vi "Begin.vi"(11 "Image Size":T1=enum."320x240") -> (0 "error out":errorcluster)   [LabVIEW 2012]
doc: "Called before other user functions, this VI is expected to open initial I/O refnums, load in file data, and do all program initialization. Notice that the <B>error out</B> terminal is simply used for data flow. Wiring it to other structures or subVIs ensures that this VI runs first."
uses:
  <vilib>/Rock Robotics/WPI/Camera/WPI_CameraImageSize.ctl
  <vilib>/Rock Robotics/WPI/DriverStation/WPI_DriverStationRobotMode2.ctl
  <vilib>/Rock Robotics/SystemInterfaces/DIO/FPGA_DIOPWMChannel.ctl
  <vilib>/Rock Robotics/WPI/Joystick/WPI_JoystickDeviceEnum.ctl
  <vilib>/Rock Robotics/SystemInterfaces/Typedef/FPGA_TypedefDigitalModule.ctl
  <vilib>/Rock Robotics/WPI/Relay/WPI_RelayDirection.ctl
  <vilib>/Rock Robotics/SystemInterfaces/DIO/FPGA_DIORelayChannel.ctl
  <vilib>/Rock Robotics/SystemInterfaces/AI/FPGA_AIChannel.ctl
  <vilib>/Rock Robotics/SystemInterfaces/AI/FPGA_AIGyroChannel.ctl
  <vilib>/Rock Robotics/SystemInterfaces/DIO/FPGA_DIOChannel.ctl
  <vilib>/Rock Robotics/WPI/Camera/WPI_CameraFrameRate.ctl
  Robot Global Data.vi
  <vilib>/Rock Robotics/WPI/MotorControl/WPI_MotorControlOpen Victor.vi
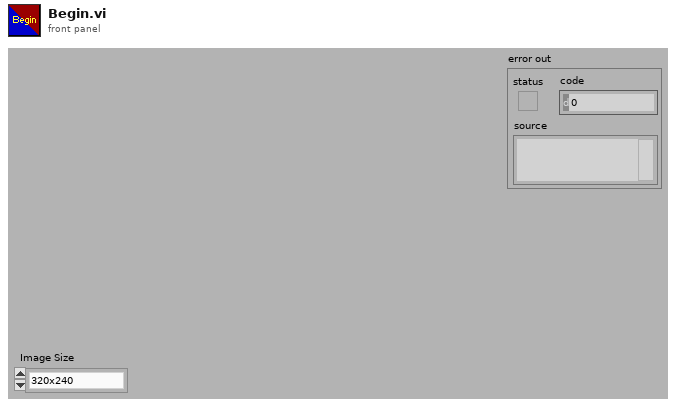
[diagram p1: front panel]
types:
  T1 = typedef "WPI_CameraImageSize.ctl" = enum16{"640x480", "320x240", "160x120"}
  T2 = typedef "FPGA_DIOChannel.ctl" = enum8{"DIO 1", "DIO 2", "DIO 3", "DIO 4", "DIO 5", "DIO 6", "DIO 7", "DIO 8", "DIO 9", "DIO 10", "DIO 11", "DIO 12", "DIO 13", "DIO 14", "Invalid"}
  T3 = typedef "FPGA_TypedefDigitalModule.ctl" = enum16{"Digital Module 1", "Digital Module 2"}
  T4 = typedef "FPGA_DIOPWMChannel.ctl" = enum8{"PWM 1", "PWM 2", "PWM 3", "PWM 4", "PWM 5", "PWM 6", "PWM 7", "PWM 8", "PWM 9", "PWM 10", "Invalid"}
  T5 = typedef "FPGA_DIORelayChannel.ctl" = enum8{"Relay 1", "Relay 2", "Relay 3", "Relay 4", "Relay 5", "Relay 6", "Relay 7", "Relay 8", "Invalid"}
  T6 = typedef "WPI_RelayDirection.ctl" = enum16{"Both directions", "Forward only", "Reverse only"}
  T7 = typedef "WPI_CameraFrameRate.ctl" = u32
  T8 = typedef "FPGA_AIChannel.ctl" = enum8{"AI 1", "AI 2", "AI 3", "AI 4", "AI 5", "AI 6", "AI 7", "AI 8", "Invalid"}
  T9 = typedef "FPGA_AIGyroChannel.ctl" = enum8{"AI 1", "AI 2", "Invalid"}
  T10 = typedef "WPI_JoystickDeviceEnum.ctl" = enum16{"USB 1", "USB 2", "USB 3", "USB 4", "Kinect 1", "Kinect 2"}
  T11 = typedef "WPI_DriverStationRobotMode2.ctl" = enum16{"Autonomous Disabled", "Autonomous Enabled", "Teleop Disabled", "Teleop Enabled", "Timeout", "Finish", "Test Disabled", "Test Enabled"}
  T12 = typedef "WPI_RelayDevRef.ctl" = cluster{"DevStatus":errorcluster, "Relay Channel":T5, "Digital Module":T3, "Relay Direction":T6}
  T13 = typedef "WPI_MotorControlDeviceRef.ctl" = cluster{"DeviceStatus":errorcluster, "Type":enum16{"PWM", "CAN"}, "PWM":cluster{"Digital Module":T3, "PWM Channel":T4, "DeadBand":T14}, "CAN":cluster{"Device Number":u8, "Control Mode":T15, "Semaphore":T16, "Max Vout":dbl}, "Invert":bool, "TransformRef":T17, "InvTransformRef":T17}
  T14 = typedef "WPI_PWMDeadband.ctl" = cluster{"Name":string, "maxPositivePwm":i32, "minPositivePwm":i32, "centerPwm":i32, "maxNegativePwm":i32, "minNegativePwm":i32, "angularRange":u16}
  T15 = typedef "WPI_CANJaguar_ControlMode.ctl" = enum8{"Percent VBus", "Current", "Speed", "Position", "Voltage"}
  T16 = typedef "Semaphore RefNum" = refnum<k1>
  T17 = typedef "WPI_PWMTransform_ConPane.ctl" = refnum<vi>
  T18 = typedef "WPI_JoystickDevRef.ctl" = cluster{"Device":T10}
  T19 = typedef "WPI_CameraDevRef.ctl" = cluster{"Camera Address":string, "CameraStatus":errorcluster, "Acquire Image Notifier":refnum<notifier>}
  T20 = typedef "WPI_ServoDeviceRef.ctl" = cluster{"DeviceStatus":errorcluster, "Digital Module":T3, "PWM Channel":T4, "DeadBand":T14}
  T21 = typedef "WPI_AnalogChannelDevRef.ctl" = cluster{"DevStatus":errorcluster, "Analog Module":T22, "Analog Channel":T8}
  T22 = typedef "FPGA_TypedefAnalogModule.ctl" = enum16{"Analog Module 1", "Analog Module 2"}
  T23 = typedef "WPI_DigitalInputDevRef.ctl" = cluster{"DevStatus":errorcluster, "DIO Channel":T2, "Digital Module":T3}
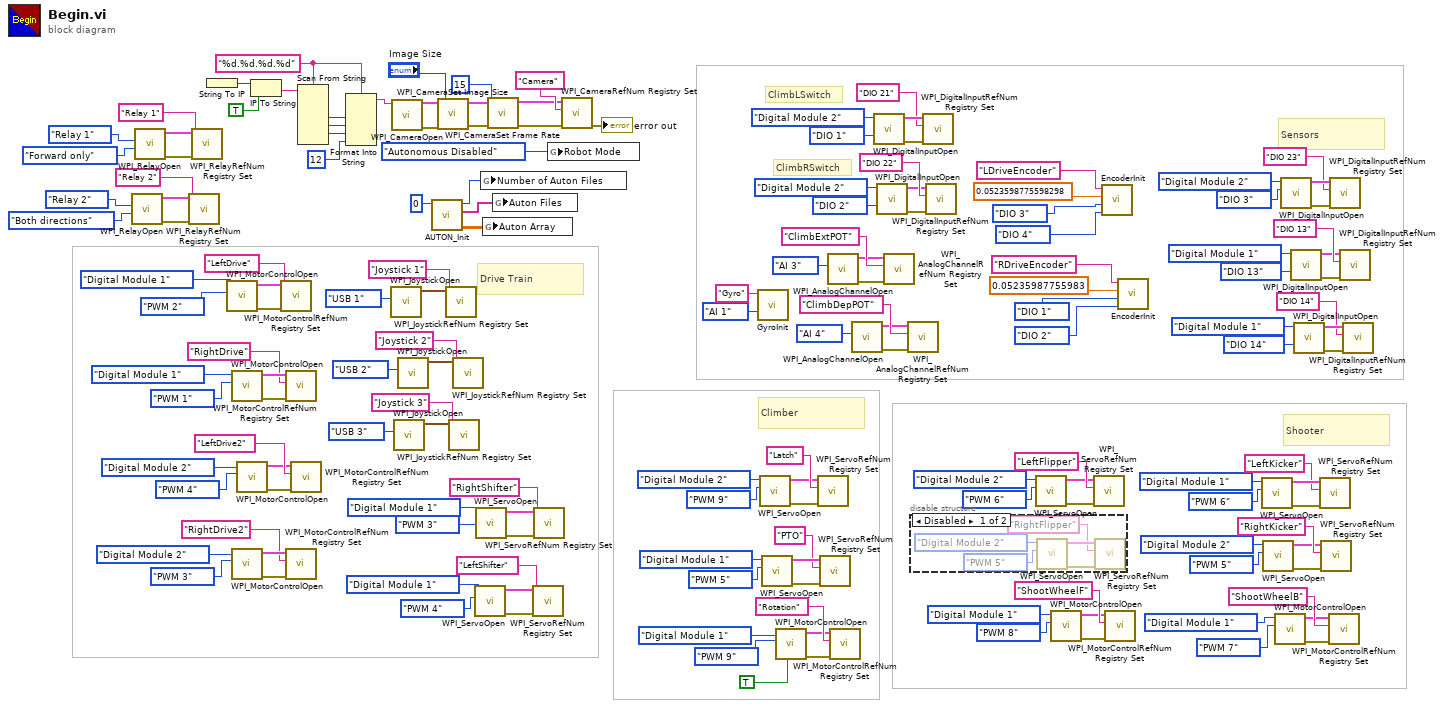
[diagram p0: block diagram]
diagram:
  w70 = "%d.%d.%d.%d" ("format string")
  # "ClimbRSwitch"
  # "ClimbLSwitch"
  # "Shooter"
  # "Drive Train"
  # "Climber"
  # "Sensors"
  n1 = call <vilib>:"WPI_RelayOpen.vi"("Relay Direction"=WPI_RelayDirection."Both directions", "Relay Channel"=FPGA_DIORelayChannel."Relay 2") -> ("error out"=w119:errorcluster, "RelayDevRef"=w120:T12)  [unwired: 8 in]
  n2 = call <vilib>:"WPI_RelayOpen.vi"("Relay Direction"=WPI_RelayDirection."Forward only", "Relay Channel"=FPGA_DIORelayChannel."Relay 1") -> ("error out"=w60:errorcluster, "RelayDevRef"=w59:T12)  [unwired: 8 in]
  n3 = call <vilib>:"WPI_RelayRefNum Registry Set.vi"("error in (no error)"=w119, "refnum name"="Relay 2", "RelayDevRef"=w120) -> ()  [unwired: 7 in, 2 out]
  n4 = call <vilib>:"WPI_RelayRefNum Registry Set.vi"("error in (no error)"=w60, "refnum name"="Relay 1", "RelayDevRef"=w59) -> ()  [unwired: 7 in, 2 out]
  n5 = String To IP() -> (0:w77:u32)  [unwired: 1 in]
  n6 = call-poly <vilib>:"WPI_MotorControlOpen.vi"("PWM Channel"=FPGA_DIOPWMChannel."PWM 2", "Digital Module (Module 1)"=FPGA_TypedefDigitalModule."Digital Module 1") -> ("error out"=w145:errorcluster, "MotorControlDeviceRef"=w146:T13)  [unwired: 8 in]
  n7 = call-poly <vilib>:"WPI_MotorControlOpen.vi"("PWM Channel"=FPGA_DIOPWMChannel."PWM 1", "Digital Module (Module 1)"=FPGA_TypedefDigitalModule."Digital Module 1") -> ("error out"=w152:errorcluster, "MotorControlDeviceRef"=w151:T13)  [unwired: 8 in]
  n8 = call-poly <vilib>:"WPI_MotorControlOpen.vi"("PWM Channel"=FPGA_DIOPWMChannel."PWM 3", "Digital Module (Module 1)"=FPGA_TypedefDigitalModule."Digital Module 2") -> ("error out"=w134:errorcluster, "MotorControlDeviceRef"=w133:T13)  [unwired: 8 in]
  n9 = call-poly <vilib>:"WPI_MotorControlOpen.vi"("PWM Channel"=FPGA_DIOPWMChannel."PWM 4", "Digital Module (Module 1)"=FPGA_TypedefDigitalModule."Digital Module 2") -> ("error out"=w125:errorcluster, "MotorControlDeviceRef"=w126:T13)  [unwired: 8 in]
  n10 = IP To String(1:TRUE ("dot notation? (F)"), 2:w77) -> (0:w75:string)
  n11 = call <vilib>:"WPI_MotorControlRefNum Registry Set.vi"("error in (no error)"=w145, "refnum name"="LeftDrive", "MotorControlDevRef"=w146) -> ()  [unwired: 7 in, 2 out]
  n12 = call <vilib>:"WPI_MotorControlRefNum Registry Set.vi"("error in (no error)"=w152, "refnum name"="RightDrive", "MotorControlDevRef"=w151) -> ()  [unwired: 7 in, 2 out]
  n13 = call <vilib>:"WPI_MotorControlRefNum Registry Set.vi"("error in (no error)"=w134, "refnum name"="RightDrive2", "MotorControlDevRef"=w133) -> ()  [unwired: 7 in, 2 out]
  n14 = call <vilib>:"WPI_MotorControlRefNum Registry Set.vi"("error in (no error)"=w125, "refnum name"="LeftDrive2", "MotorControlDevRef"=w126) -> ()  [unwired: 7 in, 2 out]
  n15 = Scan From String(format string=w70, input string=w75) -> (output 1=w74:i32, output 2=w73:i32, output 3=w72:i32)  [unwired: 7 in, 3 out]
  n16 = Format Into String(format string=w70, w74, w73, w72, 12 ("Compression")) -> (resulting string=w69:string)  [unwired: 2 in, 1 out]
  n17 = call <vilib>:"WPI_JoystickOpen.vi"("JoystickDevice"=WPI_JoystickDeviceEnum."USB 1") -> ("JoystickDevRef"=w136:T18)  [unwired: 10 in]
  n18 = call <vilib>:"WPI_CameraOpen.vi"("Camera Address"=w69) -> ("error out"=w68:errorcluster, "CameraDevRef"=w67:T19)  [unwired: 1 in, 8 out]
  n19 = call <vilib>:"WPI_JoystickOpen.vi"("JoystickDevice"=WPI_JoystickDeviceEnum."USB 3") -> ("JoystickDevRef"=w142:T18)  [unwired: 10 in]
  n20 = call <vilib>:"WPI_JoystickOpen.vi"("JoystickDevice"=WPI_JoystickDeviceEnum."USB 2") -> ("JoystickDevRef"=w141:T18)  [unwired: 10 in]
  n21 = call "AUTON_Init.vi"("Default File"=0) -> ("Auton Array"=w153:dbl[][], "Auton Files"=w154:string[], "Number of Auton Files"=w155:i64)  [unwired: 8 in]
  n22 = call <vilib>:"WPI_CameraSet Image Size.vi"("error in (no error)"=w68, "Image Size"="Image Size", "CameraDevRef"=w67) -> ("error out"=w65:errorcluster, "CameraDevRef Out"=w66:T19)  [unwired: 7 out]
  n23 = call <vilib>:"WPI_JoystickRefNum Registry Set.vi"("refnum name"="Joystick 1", "JoystickDevRef"=w136) -> ()  [unwired: 8 in, 2 out]
  n24 = call <vilib>:"WPI_JoystickRefNum Registry Set.vi"("refnum name"="Joystick 3", "JoystickDevRef"=w142) -> ()  [unwired: 8 in, 2 out]
  n25 = call <vilib>:"WPI_JoystickRefNum Registry Set.vi"("refnum name"="Joystick 2", "JoystickDevRef"=w141) -> ()  [unwired: 8 in, 2 out]
  n26 = call <vilib>:"WPI_ServoOpen.vi"("PWM Channel"=FPGA_DIOPWMChannel."PWM 4", "Digital Module (Module 1)"=FPGA_TypedefDigitalModule."Digital Module 1") -> ("error out"=w118:errorcluster, "ServoDeviceRef"=w111:T20)  [unwired: 8 in]
  n27 = call <vilib>:"WPI_ServoOpen.vi"("PWM Channel"=FPGA_DIOPWMChannel."PWM 3", "Digital Module (Module 1)"=FPGA_TypedefDigitalModule."Digital Module 1") -> ("error out"=w117:errorcluster, "ServoDeviceRef"=w116:T20)  [unwired: 8 in]
  n28 = global write "Robot Global Data.vi" "Number of Auton Files"(w155) -> ()
  n29 = global write "Robot Global Data.vi" "Auton Array"(w153) -> ()
  n30 = call <vilib>:"WPI_CameraSet Frame Rate.vi"("error in (no error)"=w65, "Frame Rate (fps)"=T7 15, "CameraDevRef"=w66) -> ("error out"=w64:errorcluster, "CameraDevRef Out"=w63:T19)  [unwired: 7 out]
  n31 = global write "Robot Global Data.vi" "Auton Files"(w154) -> ()
  n32 = call <vilib>:"WPI_ServoRefNum Registry Set.vi"("error in (no error)"=w118, "refnum name"="LeftShifter", "ServoDeviceRef"=w111) -> ()  [unwired: 7 in, 2 out]
  n33 = call <vilib>:"WPI_ServoRefNum Registry Set.vi"("error in (no error)"=w117, "refnum name"="RightShifter", "ServoDeviceRef"=w116) -> ()  [unwired: 7 in, 2 out]
  n34 = global write "Robot Global Data.vi" "Robot Mode"(WPI_DriverStationRobotMode2."Autonomous Disabled" ("Robot Mode")) -> ()
  n35 = call <vilib>:"WPI_CameraRefNum Registry Set.vi"("error in (no error)"=w64, "refnum name"="Camera", "CameraDevRef"=w63) -> ("error out"=→"error out":errorcluster)  [unwired: 8 out]
  n36 = call "GyroInit.vi"("refnum name"="Gyro", "Analog Channel"=FPGA_AIGyroChannel."AI 1") -> ()  [unwired: 8 in]
  n37 = call <vilib>:"WPI_ServoOpen.vi"("PWM Channel"=FPGA_DIOPWMChannel."PWM 9", "Digital Module (Module 1)"=FPGA_TypedefDigitalModule."Digital Module 2") -> ("error out"=w52:errorcluster, "ServoDeviceRef"=w53:T20)  [unwired: 8 in]
  n38 = call <vilib>:"WPI_ServoOpen.vi"("PWM Channel"=FPGA_DIOPWMChannel."PWM 5", "Digital Module (Module 1)"=FPGA_TypedefDigitalModule."Digital Module 1") -> ("error out"=w96:errorcluster, "ServoDeviceRef"=w95:T20)  [unwired: 8 in]
  n39 = call-poly <vilib>:"WPI_MotorControlOpen.vi"("Invert"=TRUE, "PWM Channel"=FPGA_DIOPWMChannel."PWM 9", "Digital Module (Module 1)"=FPGA_TypedefDigitalModule."Digital Module 1") -> ("error out"=w101:errorcluster, "MotorControlDeviceRef"=w100:T13)  [unwired: 7 in]
  n40 = call <vilib>:"WPI_ServoRefNum Registry Set.vi"("error in (no error)"=w52, "refnum name"="Latch", "ServoDeviceRef"=w53) -> ()  [unwired: 7 in, 2 out]
  n41 = call <vilib>:"WPI_ServoRefNum Registry Set.vi"("error in (no error)"=w96, "refnum name"="PTO", "ServoDeviceRef"=w95) -> ()  [unwired: 7 in, 2 out]
  n42 = call <vilib>:"WPI_AnalogChannelOpen.vi"("Analog Channel"=FPGA_AIChannel."AI 3") -> ("error out"=w80:errorcluster, "AIDeviceRef"=w81:T21)  [unwired: 9 in]
  n43 = call <vilib>:"WPI_MotorControlRefNum Registry Set.vi"("error in (no error)"=w101, "refnum name"="Rotation", "MotorControlDevRef"=w100) -> ()  [unwired: 7 in, 2 out]
  n44 = call <vilib>:"WPI_AnalogChannelOpen.vi"("Analog Channel"=FPGA_AIChannel."AI 4") -> ("error out"=w105:errorcluster, "AIDeviceRef"=w106:T21)  [unwired: 9 in]
  n45 = call <vilib>:"WPI_DigitalInputOpen.vi"("DIO Channel"=FPGA_DIOChannel."DIO 1", "Digital Module (Module 1)"=FPGA_TypedefDigitalModule."Digital Module 2") -> ("error out"=w2:errorcluster, "DigitalInputDevRef"=w3:T23)  [unwired: 8 in]
  n46 = call <vilib>:"WPI_DigitalInputOpen.vi"("DIO Channel"=FPGA_DIOChannel."DIO 2", "Digital Module (Module 1)"=FPGA_TypedefDigitalModule."Digital Module 2") -> ("error out"=w9:errorcluster, "DigitalInputDevRef"=w8:T23)  [unwired: 8 in]
  n47 = call <vilib>:"WPI_AnalogChannelRefNum Registry Set.vi"("error in (no error)"=w80, "refnum name"="ClimbExtPOT", "AIDeviceRef"=w81) -> ()  [unwired: 7 in, 2 out]
  n48 = call <vilib>:"WPI_AnalogChannelRefNum Registry Set.vi"("error in (no error)"=w105, "refnum name"="ClimbDepPOT", "AIDeviceRef"=w106) -> ()  [unwired: 7 in, 2 out]
  n49 = disable-structure shown="Disabled" {
    frame Disabled {
      n50 = call <vilib>:"WPI_ServoOpen.vi"("PWM Channel"=FPGA_DIOPWMChannel."PWM 5", "Digital Module (Module 1)"=FPGA_TypedefDigitalModule."Digital Module 2") -> ("error out"=w162:errorcluster, "ServoDeviceRef"=w161:T20)  [unwired: 8 in]
      n51 = call <vilib>:"WPI_ServoRefNum Registry Set.vi"("error in (no error)"=w162, "refnum name"="RightFlipper", "ServoDeviceRef"=w161) -> ()  [unwired: 7 in, 2 out]
    }
    frame Enabled {
    }
  }
  n52 = call <vilib>:"WPI_DigitalInputRefNum Registry Set.vi"("error in (no error)"=w2, "refnum name"="DIO 21", "DigitalInputDevRef"=w3) -> ()  [unwired: 7 in, 2 out]
  n53 = call <vilib>:"WPI_DigitalInputRefNum Registry Set.vi"("error in (no error)"=w9, "refnum name"="DIO 22", "DigitalInputDevRef"=w8) -> ()  [unwired: 7 in, 2 out]
  n54 = call <vilib>:"WPI_ServoOpen.vi"("PWM Channel"=FPGA_DIOPWMChannel."PWM 6", "Digital Module (Module 1)"=FPGA_TypedefDigitalModule."Digital Module 2") -> ("error out"=w36:errorcluster, "ServoDeviceRef"=w37:T20)  [unwired: 8 in]
  n55 = call-poly <vilib>:"WPI_MotorControlOpen.vi"("PWM Channel"=FPGA_DIOPWMChannel."PWM 8", "Digital Module (Module 1)"=FPGA_TypedefDigitalModule."Digital Module 1") -> ("error out"=w47:errorcluster, "MotorControlDeviceRef"=w48:T13)  [unwired: 8 in]
  n56 = call <vilib>:"WPI_ServoRefNum Registry Set.vi"("error in (no error)"=w36, "refnum name"="LeftFlipper", "ServoDeviceRef"=w37) -> ()  [unwired: 7 in, 2 out]
  n57 = call "EncoderInit.vi"("refnum name"="LDriveEncoder", "DistancePerCount"=0.0523598775598298, "DIO Channel"=FPGA_DIOChannel."DIO 3", "DIO Channel 2"=FPGA_DIOChannel."DIO 4") -> ()  [unwired: 7 in]
  n58 = call <vilib>:"WPI_MotorControlRefNum Registry Set.vi"("error in (no error)"=w47, "refnum name"="ShootWheelF", "MotorControlDevRef"=w48) -> ()  [unwired: 7 in, 2 out]
  n59 = call "EncoderInit.vi"("refnum name"="RDriveEncoder", "DistancePerCount"=0.05235987755983, "DIO Channel"=FPGA_DIOChannel."DIO 1", "DIO Channel 2"=FPGA_DIOChannel."DIO 2") -> ()  [unwired: 7 in]
  n60 = call <vilib>:"WPI_ServoOpen.vi"("PWM Channel"=FPGA_DIOPWMChannel."PWM 6", "Digital Module (Module 1)"=FPGA_TypedefDigitalModule."Digital Module 1") -> ("error out"=w31:errorcluster, "ServoDeviceRef"=w30:T20)  [unwired: 8 in]
  n61 = call <vilib>:"WPI_ServoOpen.vi"("PWM Channel"=FPGA_DIOPWMChannel."PWM 5", "Digital Module (Module 1)"=FPGA_TypedefDigitalModule."Digital Module 2") -> ("error out"=w26:errorcluster, "ServoDeviceRef"=w32:T20)  [unwired: 8 in]
  n62 = call-poly <vilib>:"WPI_MotorControlOpen.vi"("PWM Channel"=FPGA_DIOPWMChannel."PWM 7", "Digital Module (Module 1)"=FPGA_TypedefDigitalModule."Digital Module 1") -> ("error out"=w43:errorcluster, "MotorControlDeviceRef"=w42:T13)  [unwired: 8 in]
  n63 = call <vilib>:"WPI_DigitalInputOpen.vi"("DIO Channel"=FPGA_DIOChannel."DIO 3", "Digital Module (Module 1)"=FPGA_TypedefDigitalModule."Digital Module 2") -> ("error out"=w11:errorcluster, "DigitalInputDevRef"=w14:T23)  [unwired: 8 in]
  n64 = call <vilib>:"WPI_DigitalInputOpen.vi"("DIO Channel"=FPGA_DIOChannel."DIO 13", "Digital Module (Module 1)"=FPGA_TypedefDigitalModule."Digital Module 1") -> ("error out"=w24:errorcluster, "DigitalInputDevRef"=w23:T23)  [unwired: 8 in]
  n65 = call <vilib>:"WPI_DigitalInputOpen.vi"("DIO Channel"=FPGA_DIOChannel."DIO 14", "Digital Module (Module 1)"=FPGA_TypedefDigitalModule."Digital Module 1") -> ("error out"=w17:errorcluster, "DigitalInputDevRef"=w18:T23)  [unwired: 8 in]
  n66 = call <vilib>:"WPI_ServoRefNum Registry Set.vi"("error in (no error)"=w31, "refnum name"="LeftKicker", "ServoDeviceRef"=w30) -> ()  [unwired: 7 in, 2 out]
  n67 = call <vilib>:"WPI_ServoRefNum Registry Set.vi"("error in (no error)"=w26, "refnum name"="RightKicker", "ServoDeviceRef"=w32) -> ()  [unwired: 7 in, 2 out]
  n68 = call <vilib>:"WPI_MotorControlRefNum Registry Set.vi"("error in (no error)"=w43, "refnum name"="ShootWheelB", "MotorControlDevRef"=w42) -> ()  [unwired: 7 in, 2 out]
  n69 = call <vilib>:"WPI_DigitalInputRefNum Registry Set.vi"("error in (no error)"=w11, "refnum name"="DIO 23", "DigitalInputDevRef"=w14) -> ()  [unwired: 7 in, 2 out]
  n70 = call <vilib>:"WPI_DigitalInputRefNum Registry Set.vi"("error in (no error)"=w24, "refnum name"="DIO 13", "DigitalInputDevRef"=w23) -> ()  [unwired: 7 in, 2 out]
  n71 = call <vilib>:"WPI_DigitalInputRefNum Registry Set.vi"("error in (no error)"=w17, "refnum name"="DIO 14", "DigitalInputDevRef"=w18) -> ()  [unwired: 7 in, 2 out]
